vi "Filter Data.vi"(10 "kp":dbl, 11 "Error":dbl) -> (2 "Chart Data":dbl, 3 "Correction Out":dbl)   [LabVIEW 2025]
uses:
  <vilib>/ptbypt/NI_PtbyPt.lvlib
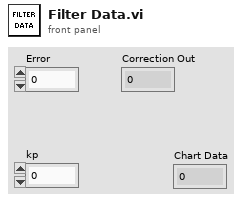
[diagram p1: front panel]
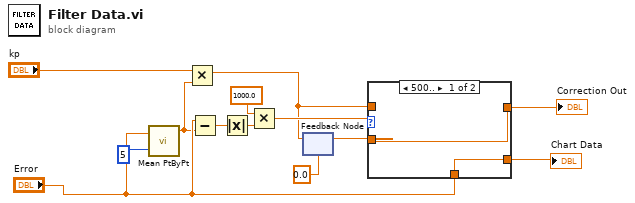
[diagram p0: block diagram]
diagram:
  n1 = call <vilib>:"Mean PtByPt.vi"("x"="Error", "sample length"=5) -> ("mean"=w1:dbl)  [unwired: 2 in, 1 out]
  n2 = Multiply(x="kp", y=w1) -> (x*y=w2:dbl)
  n3 = Subtract(x="Error", y=w1) -> (x-y=w10:dbl)
  n4 = Absolute Value(x=w10) -> (abs(x)=w11:dbl)
  n5 = Multiply(x=1000.0, y=w11) -> (x*y=w13:dbl)
  n6 = feedback #1(0.0 ("f")) -> (w6:dbl)
  n7 = feedback-in #1(w2) -> ()
  n8 = case shown="500.." w13 {
    tunnel: w2 -> [_ w16]
    tunnel: [w15 w16] -> w7
    tunnel: w6 -> [w15 _]
    tunnel: "Error" -> [w14 _]
    tunnel: [w14 _] -> w8
    frame 500.. {
    }
    frame Default {
    }
  }
  "Chart Data" <- w8
  "Correction Out" <- w7
